vi "Create Command.vi"(8 "error in":errorcluster, 11 "RequestData":T1={"Mode"="sdg", "Operator"="o", "SerialNo"="s", "HuNo"="h", "MaterialCode"="mm", "PackingInstructions"="p", "ProductionVersion"="pp"}) -> (0 "error out":errorcluster)   [LabVIEW 2023, in "MES.lvlib"]
uses:
  MES.lvlib
  <vilib>/xml/Load XML File.vi
  <vilib>/xml/Close Reference(Node).vi
  <vilib>/xml/Close Reference(NdList).vi
  <resource>/objmgr/DOMUserDefRef.rc
  <vilib>/xml/NI_XML.lvlib
  RequestData.ctl
panel:
  out "Parse Errors":string
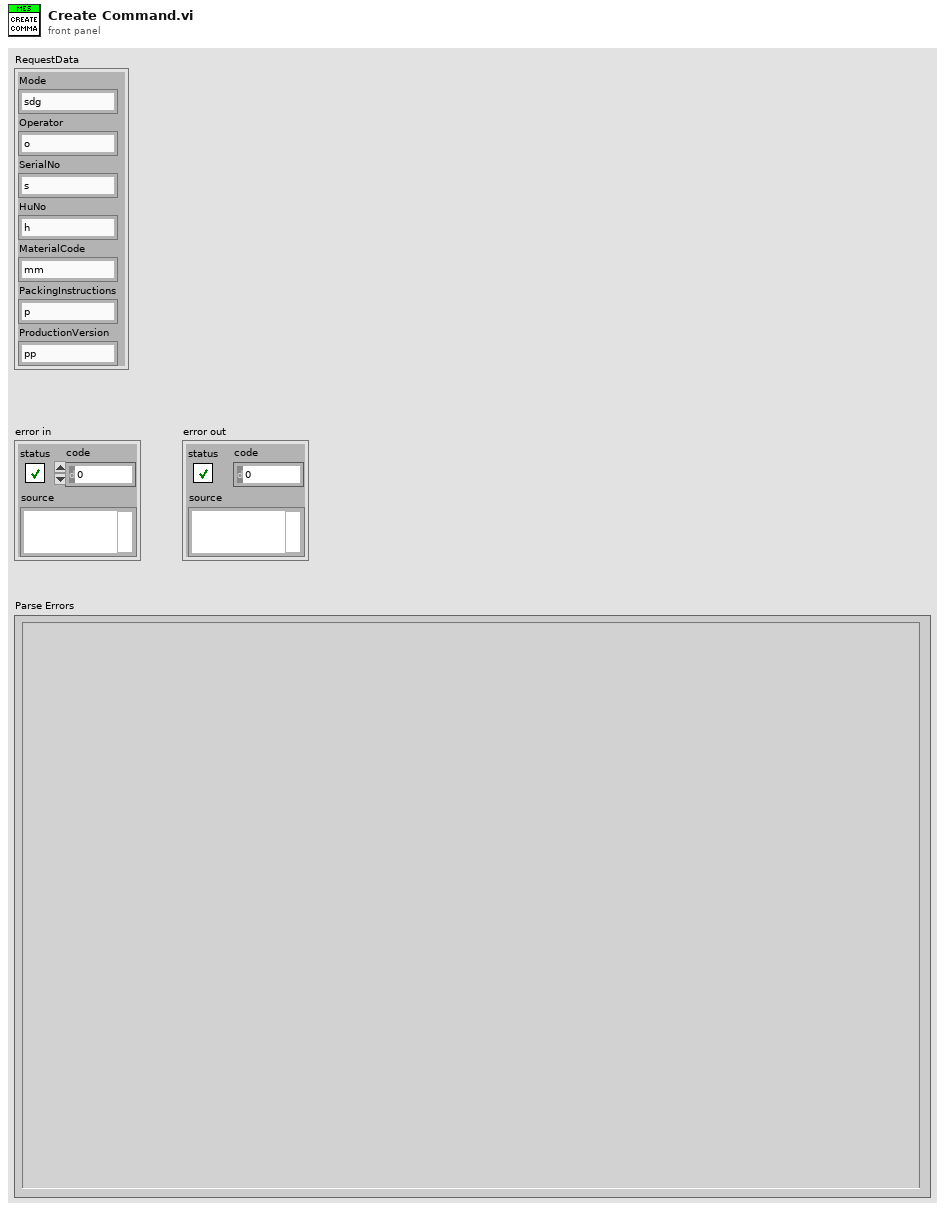
[diagram p1: front panel]
types:
  T1 = typedef "RequestData.ctl" = cluster{"Mode":string, "Operator":string, "SerialNo":string, "HuNo":string, "MaterialCode":string, "PackingInstructions":string, "ProductionVersion":string}
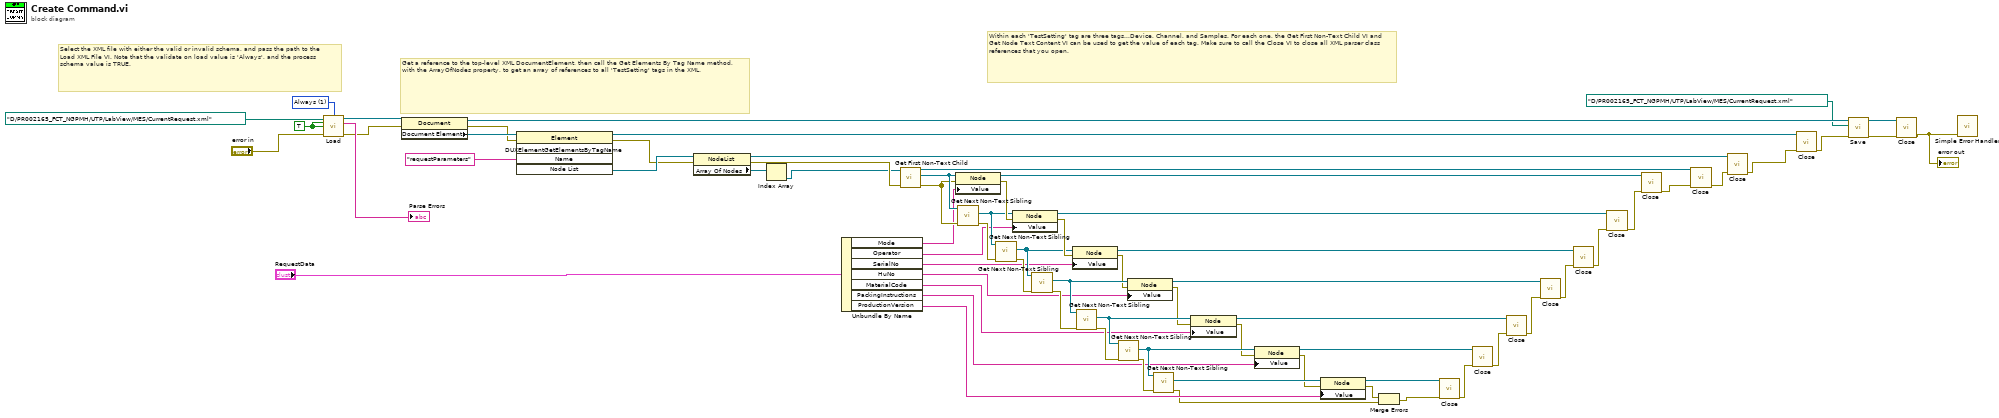
[diagram p0: block diagram]
diagram:
  w70 = 1 items=["Never", "Always", "Auto"] ("Validate On Load")
  w57 = TRUE ("Do Namespaces")
  # "Within each 'TestSetting' tag are three tags...Device, Channel, and Samples. For each one, the Get First Non-Text Child VI and Get Node Text Content VI can be used to get the value of each tag. Make sure to call the Close VI to close all XML parser class references that you open."
  # "Get a reference to the top-level XML DocumentElement, then call the Get Elements By Tag Name method, with the ArrayOfNodes property, to get an array of references to all 'TestSetting' tags in the XML."
  # "Select the XML file with either the valid or invalid schema, and pass the path to the Load XML File VI. Note that the validate on load value is 'Always', and the process schema value is TRUE."
  n1 = call-poly <vilib>:"Load.vi"("path to XML document"=path "D:/PR002165_FCT_NGPMH/UTP/LabView/MES/CurrentRequest.xml" ("file path (use dialog)"), "validate on load (Auto)"=w70, "process namespaces (False)"=w57, "process schema (False)"=w57, "error in (no error)"="error in") -> ("DOM document out"=w59:refnum<k20>, "parse errors"=→"Parse Errors":string, "error out"=w58:errorcluster)  [unwired: 2 in, 6 out]
  n2 = property class="Document"(reference=w59, error in=w58) -> (reference out=w7:refnum<k20>, error out=w66:errorcluster, "Document Element"=w67:refnum<k20>)
  n3 = invoke class="Element" method="DUXElementGetElementsByTagName"(reference=w67, error in=w66, "Name"="requestParameters" ("Node Name")) -> (reference out=w60:refnum<k20>, error out=w64:errorcluster, "Node List"=w65:refnum<k20>)  [unwired: 2 in, 2 out]
  n4 = property class="NodeList"(reference=w65, error in=w64) -> (reference out=w63:refnum<k20>, error out=w62:errorcluster, "Array Of Nodes"=w54:refnum<k20>[])
  n5 = Index Array(array=w54) -> (element=w53:refnum<k20>)  [unwired: 1 in]
  n6 = Unbundle By Name("RequestData") -> ("Mode"=w29:string, "Operator"=w28:string, "SerialNo"=w27:string, "HuNo"=w26:string, "MaterialCode"=w25:string, "PackingInstructions"=w24:string, "ProductionVersion"=w23:string)
  n7 = call <vilib>:"Get First Non-Text Child.vi"("error in (no error)"=w62, "node in"=w53) -> ("error out"=w47:errorcluster, "child node"=w48:refnum<k20>, "node out"=w51:refnum<k20>)  [unwired: 7 out]
  n8 = property class="Node"(reference=w48, error in=w47, "Value"=w29) -> (reference out=w22:refnum<k20>, error out=w46:errorcluster)
  n9 = call <vilib>:"Get Next Non-Text Sibling.vi"("error in (no error)"=w47, "node in"=w48) -> ("error out"=w45:errorcluster, "sibling node"=w42:refnum<k20>)  [unwired: 8 out]
  n10 = call <vilib>:"Get Next Non-Text Sibling.vi"("error in (no error)"=w45, "node in"=w42) -> ("error out"=w33:errorcluster, "sibling node"=w43:refnum<k20>)  [unwired: 8 out]
  n11 = property class="Node"(reference=w42, error in=w46, "Value"=w28) -> (reference out=w21:refnum<k20>, error out=w44:errorcluster)
  n12 = call <vilib>:"Get Next Non-Text Sibling.vi"("error in (no error)"=w33, "node in"=w43) -> ("error out"=w32:errorcluster, "sibling node"=w41:refnum<k20>)  [unwired: 8 out]
  n13 = property class="Node"(reference=w43, error in=w44, "Value"=w27) -> (reference out=w20:refnum<k20>, error out=w37:errorcluster)
  n14 = call <vilib>:"Get Next Non-Text Sibling.vi"("error in (no error)"=w32, "node in"=w41) -> ("error out"=w31:errorcluster, "sibling node"=w40:refnum<k20>)  [unwired: 8 out]
  n15 = call <vilib>:"Get Next Non-Text Sibling.vi"("error in (no error)"=w31, "node in"=w40) -> ("error out"=w30:errorcluster, "sibling node"=w39:refnum<k20>)  [unwired: 8 out]
  n16 = property class="Node"(reference=w41, error in=w37, "Value"=w26) -> (reference out=w19:refnum<k20>, error out=w36:errorcluster)
  n17 = call <vilib>:"Get Next Non-Text Sibling.vi"("error in (no error)"=w30, "node in"=w39) -> ("error out"=w8:errorcluster, "sibling node"=w38:refnum<k20>)  [unwired: 8 out]
  n18 = property class="Node"(reference=w40, error in=w36, "Value"=w25) -> (reference out=w15:refnum<k20>, error out=w35:errorcluster)
  n19 = property class="Node"(reference=w39, error in=w35, "Value"=w24) -> (reference out=w16:refnum<k20>, error out=w34:errorcluster)
  n20 = property class="Node"(reference=w38, error in=w34, "Value"=w23) -> (reference out=w18:refnum<k20>, error out=w10:errorcluster)
  n21 = Merge Errors(w10, w8) -> (w9:errorcluster)
  n22 = call-poly <vilib>:"Close.vi"("error in (no error)"=w9, "node"=w18) -> ("error out"=w17:errorcluster)  [unwired: 7 out]
  n23 = call-poly <vilib>:"Close.vi"("error in (no error)"=w17, "node"=w16) -> ("error out"=w14:errorcluster)  [unwired: 7 out]
  n24 = call-poly <vilib>:"Close.vi"("error in (no error)"=w14, "node"=w15) -> ("error out"=w13:errorcluster)  [unwired: 7 out]
  n25 = call-poly <vilib>:"Close.vi"("error in (no error)"=w13, "node"=w19) -> ("error out"=w12:errorcluster)  [unwired: 7 out]
  n26 = call-poly <vilib>:"Close.vi"("error in (no error)"=w12, "node"=w20) -> ("error out"=w11:errorcluster)  [unwired: 7 out]
  n27 = call-poly <vilib>:"Close.vi"("error in (no error)"=w11, "node"=w21) -> ("error out"=w52:errorcluster)  [unwired: 7 out]
  n28 = call-poly <vilib>:"Close.vi"("error in (no error)"=w52, "node"=w22) -> ("error out"=w50:errorcluster)  [unwired: 7 out]
  n29 = call-poly <vilib>:"Close.vi"("error in (no error)"=w50, "node"=w51) -> ("error out"=w49:errorcluster)  [unwired: 7 out]
  n30 = call-poly <vilib>:"Close.vi"("error in (no error)"=w49, "node list"=w63) -> ("error out"=w61:errorcluster)  [unwired: 7 out]
  n31 = call-poly <vilib>:"Close.vi"("error in (no error)"=w61, "node"=w60) -> ("error out"=w5:errorcluster)  [unwired: 7 out]
  n32 = call <vilib>:"Save.vi"("error in (no error)"=w5, "XML file path"=path "D:/PR002165_FCT_NGPMH/UTP/LabView/MES/CurrentRequest.xml" ("file path (use dialog)"), "DOM document in"=w7) -> ("error out"=w4:errorcluster, "DOM document out"=w6:refnum<k20>)  [unwired: 6 in, 1 out]
  n33 = call-poly <vilib>:"Close.vi"("error in (no error)"=w4, "node"=w6) -> ("error out"=w1:errorcluster)  [unwired: 7 out]
  "error out" <- w1
  n34 = call <vilib>:"Simple Error Handler.vi"("error in (no error)"=w1) -> ()  [unwired: 4 in, 5 out]
